vi "User_Info.vi"() -> ()   [LabVIEW 2020]
panel:
  in  "Change User":bool caption="切换用户"
  in  "User Manage":bool
  in  "Change Password":bool
  in  "User_Right":u16(ring) caption="权    限" items=["原厂管理员", "超级管理员", "操作者"]
  in  "User_Name":string caption="用户名"
  # "用户信息"
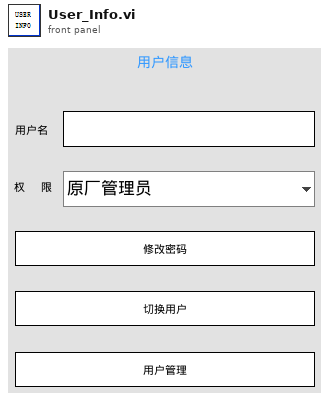
[diagram p1: front panel]
types:
  T1 = typedef "User_Info.ctl" = cluster{"Name":string, "Password":string, "User_Right":u16, "Debuger?":bool, "Manager?":bool, "User_Remember_Name":bool, "User_Remember_PW":bool, "User_Right_String":string, "Null?":bool, "Language":string}
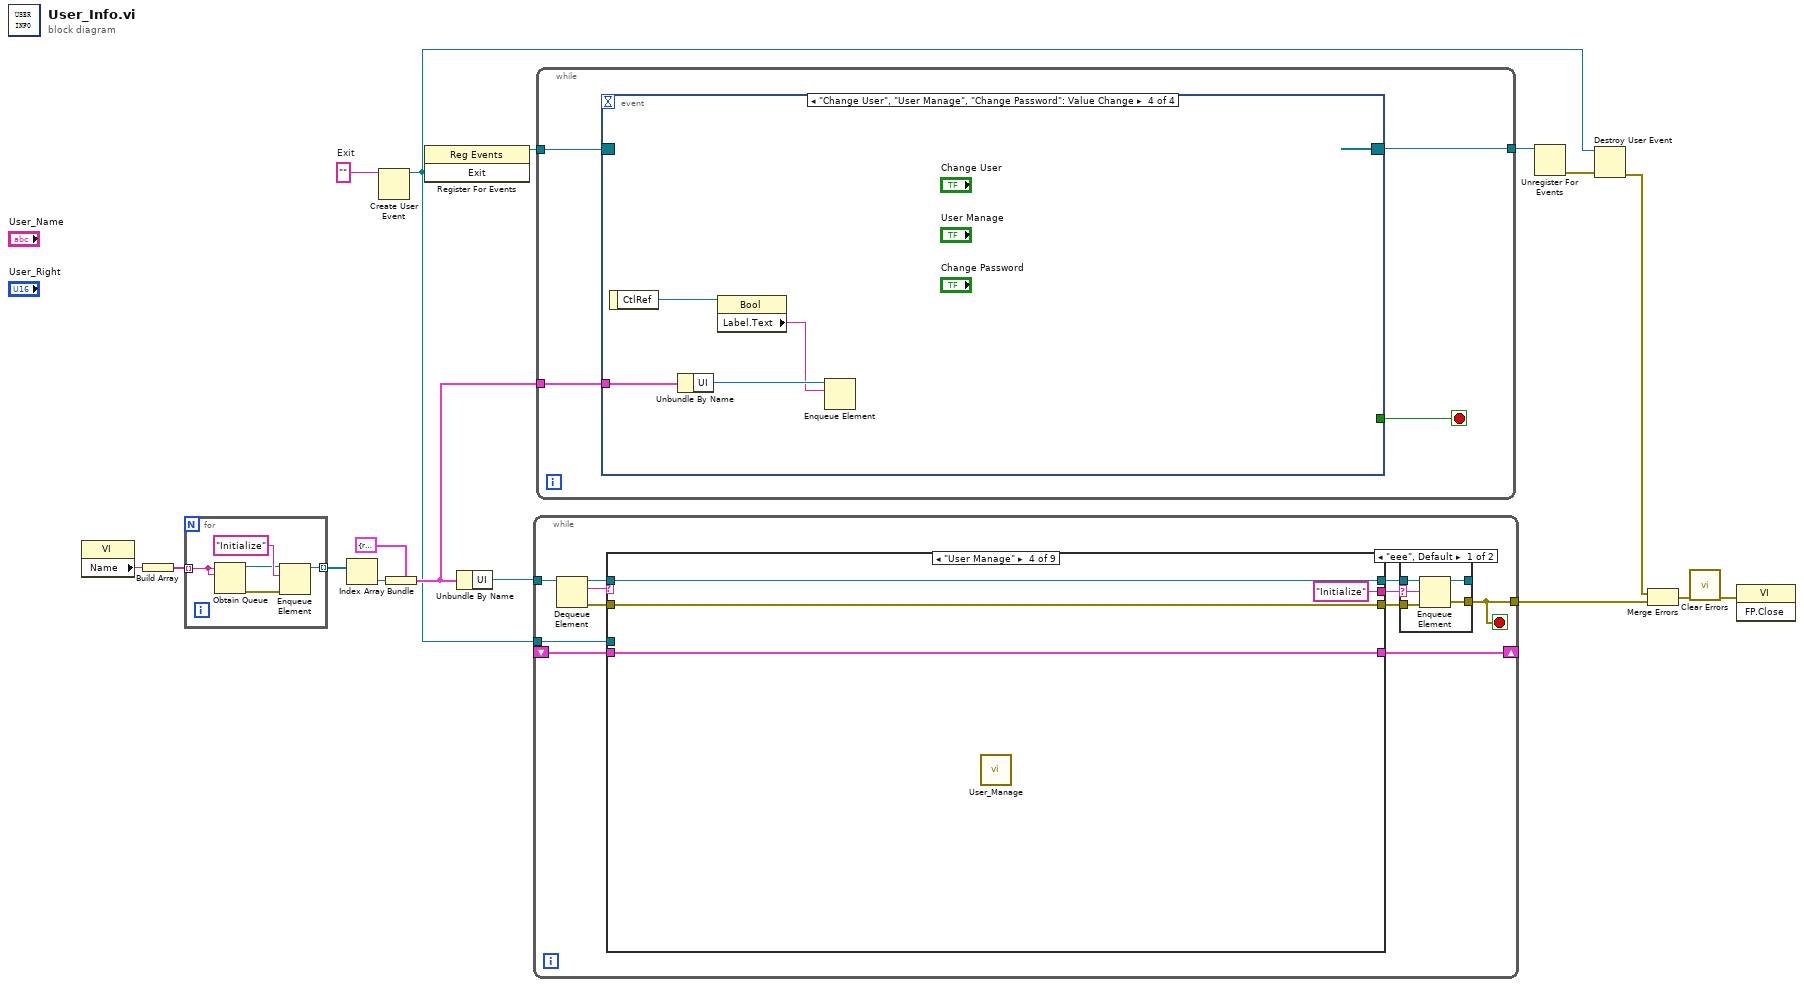
[diagram p0: block diagram]
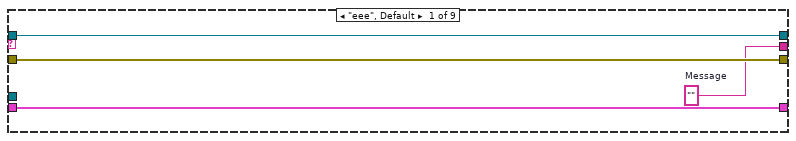
[diagram p3: hidden frame]
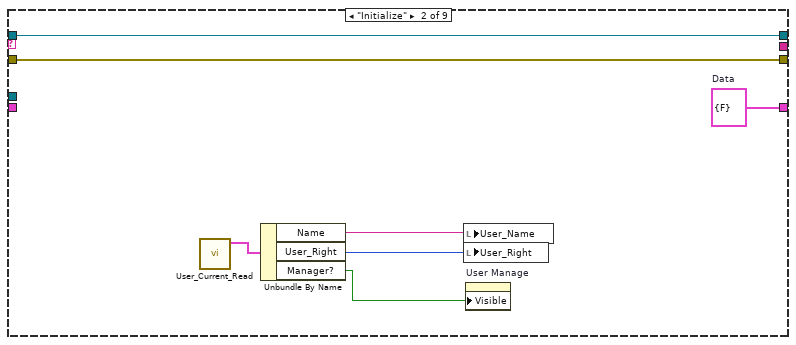
[diagram p4: hidden frame]
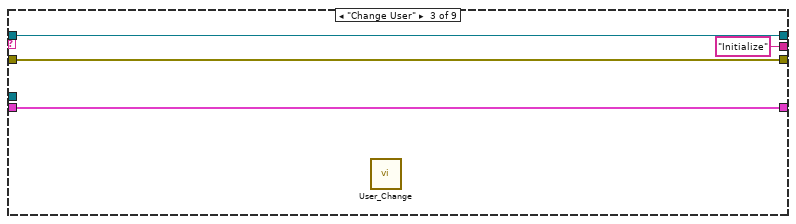
[diagram p5: hidden frame]
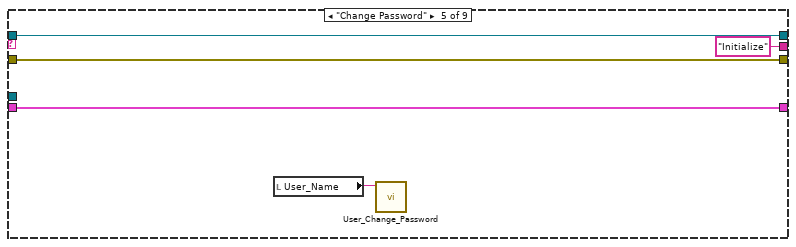
[diagram p6: hidden frame]
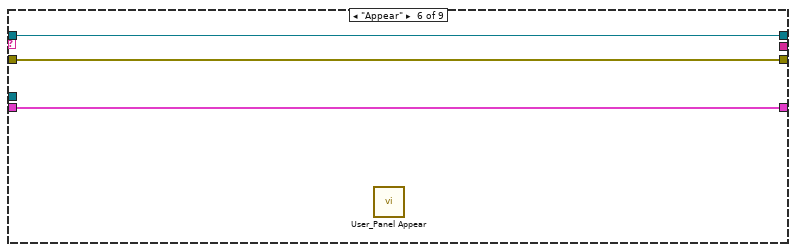
[diagram p7: hidden frame]
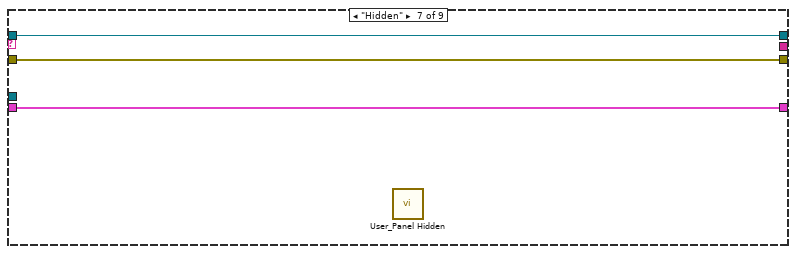
[diagram p8: hidden frame]
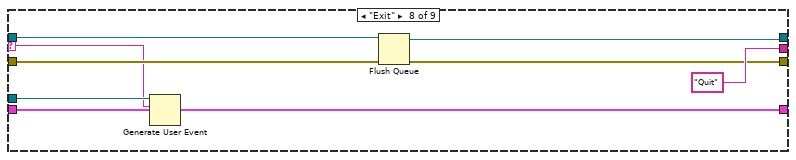
[diagram p9: hidden frame]
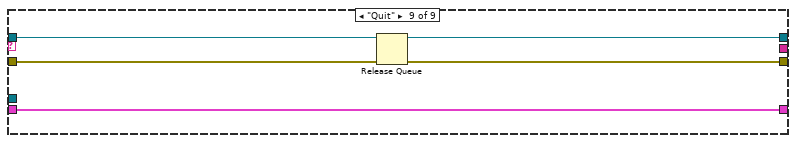
[diagram p10: hidden frame]
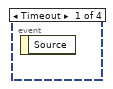
[diagram p11: hidden frame]
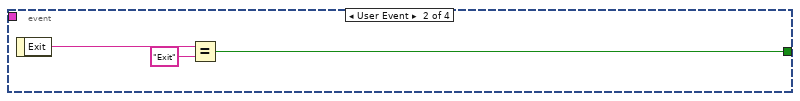
[diagram p12: hidden frame]
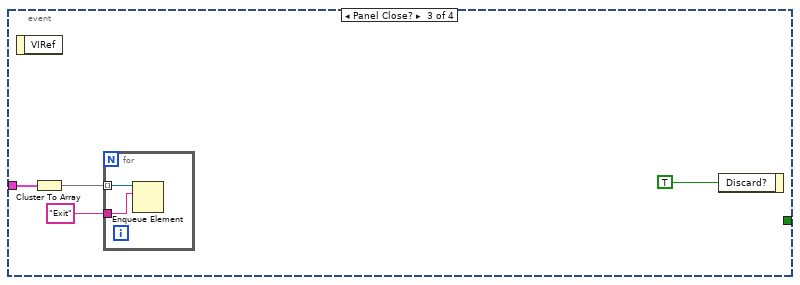
[diagram p13: hidden frame]
diagram:
  w2 = ""  # Exit
  n1 = property class="VI"() -> ("Name"=w12:string)  [unwired: 2 in, 2 out]
  n2 = Build Array(w12) -> (w13:string[])
  n3 = for {
    tunnel: w13 -> [w17] mode=indexing
    tunnel: [w18] -> w7 mode=indexing
    n4 = Obtain Queue(name (unnamed)=w17, element data type=w17) -> (queue out=w20:refnum<queue>, error out=w19:errorcluster)  [unwired: 3 in, 1 out]
    n5 = Enqueue Element(queue=w20, element="Initialize" ("元素"), error in (no error)=w19) -> (queue out=w18:refnum<queue>)  [unwired: 1 in, 2 out]
  }
  n6 = Index Array(array=w7) -> (element=w10:refnum<queue>)  [unwired: 1 in]
  n7 = Create User Event(user event datatype=w2) -> (user event=w6:refnum<user-event>)  [unwired: 1 in, 1 out]
  n8 = Bundle(cluster=cluster{"UI":refnum<queue>} {"UI"=refnum}, "UI"=w10) -> (w11:cluster{"UI":refnum<queue>})
  n9 = register-events(w6) -> (reference out=w3:refnum<event-registration>)  [unwired: 2 in, 1 out]
  n10 = Unbundle By Name(w11) -> ("UI"=w8:refnum<queue>)
  n11 = while {
    tunnel: w8 -> [w32]
    tunnel: [w22] -> w15
    shift-right: [w26] -> _
    shift-left: _ -> [w25]
    tunnel: w6 -> [w24]
    stop <- w22 stop-if-true
    n12 = Dequeue Element(queue=w32) -> (queue out=w31:refnum<queue>, element=w23:string, error out=w28:errorcluster)  [unwired: 2 in, 1 out]
    n13 = case shown="\"User Manage\"" w23 {
      selector: w23 -> [_ _ _ _ _ _ _ w70 _]
      tunnel: w31 -> [w43 w50 w54 w58 w63 w66 w69 w75 w81]
      tunnel: [w43 w50 w54 w58 w63 w66 w69 w74 w81] -> w30
      tunnel: [w42 w49 w53 w57 w62 w65 w68 w73 w78] -> w29
      tunnel: w28 -> [w42 w49 w53 w57 w62 w65 w68 w72 w80]
      tunnel: [w41 _ "Initialize" ("Message") "Initialize" ("Message") "Initialize" ("Message") _ _ "Quit" ("Message") _] -> w27
      tunnel: [w40 w48 w52 w56 w61 w64 w67 w77 w79] -> w26
      tunnel: w25 -> [w40 _ w52 w56 w61 w64 w67 w77 w79]
      tunnel: w24 -> [_ _ _ _ _ _ _ w71 _]
      frame "eee", Default {
        w41 = ""  # Message
      }
      frame "Initialize" {
        w48 = cluster{"Data":bool} {"Data"=FALSE}  # Data
        n14 = call "User_Current_Read.vi"() -> ("User_Info"=w47:T1)  [unwired: 10 in, 1 out]
        n15 = Unbundle By Name(w47) -> ("Name"=w46:string, "User_Right"=w45:u16, "Manager?"=w44:bool)
        n16 = local write "User_Name"(w46) -> ()
        n17 = local write "User_Right"(w45) -> ()
        n18 = property on="User Manage" class="Bool"("Visible"=w44) -> ()  [unwired: 2 in, 2 out]
      }
      frame "Change User" {
        n19 = call "User_Change.vi"() -> ()  [unwired: 12 in]
      }
      frame "User Manage" {
        n20 = call "User_Manage.vi"() -> ()  [unwired: 12 in]
      }
      frame "Change Password" {
        n21 = local read "User_Name"() -> (w59:string)
        n22 = call "User_Change_Password.vi"("User_Name"=w59) -> ()  [unwired: 11 in]
      }
      frame "Appear" {
        n23 = call "User_Panel Appear.vi"() -> ()  [unwired: 11 in, 1 out]
      }
      frame "Hidden" {
        n24 = call "User_Panel Hidden.vi"() -> ()  [unwired: 11 in, 1 out]
      }
      frame "Exit" {
        n25 = Generate User Event(user event=w71, event data cluster=w70) -> ()  [unwired: 2 in, 2 out]
        n26 = Flush Queue(queue=w75, error in (no error)=w72) -> (queue out=w74:refnum<queue>, error out=w73:errorcluster)  [unwired: 1 out]
      }
      frame "Quit" {
        n27 = Release Queue(queue=w81, error in (no error)=w80) -> (error out=w78:errorcluster)  [unwired: 1 in, 2 out]
      }
    }
    n28 = case shown="\"eee\", Default" w27 {
      selector: w27 -> [w33 _]
      tunnel: w30 -> [w37 w39]
      tunnel: w29 -> [w36 w38]
      tunnel: [w35 w38] -> w22
      tunnel: [w34 w39] -> _
      frame "eee", Default {
        n29 = Enqueue Element(queue=w37, element=w33, error in (no error)=w36) -> (queue out=w34:refnum<queue>, error out=w35:errorcluster)  [unwired: 1 in, 1 out]
      }
      frame "" {
      }
    }
  }
  n30 = while {
    tunnel: w3 -> [w84]
    tunnel: [w83] -> w5
    tunnel: w11 -> [w82]
    stop <- w85 stop-if-true
    n31 = event shown="[3] \"Change User\", \"User Manage\", \"Change Password\": Value Change" {
      selector: w84 -> [_ _ _ _]
      dyn-events: [_ _ _ _] -> w83
      timeout: _ -> [_ _ _ _]
      tunnel: [_ w87 _ _] -> w85
      tunnel: w82 -> [_ _ w91 w98]
      event Timeout {
        n32 = event-data() -> ()  [unwired: 1 in, 1 out]
      }
      event User Event {
        n33 = event-data() -> ("Exit"=w88:string)  [unwired: 1 in]
        n34 = Equal?(x=w88, y="Exit") -> (x = y?=w87:bool)
      }
      event Panel Close? {
        n35 = event-data() -> ()  [unwired: 1 in, 1 out]
        n36 = Cluster To Array(cluster=w91) -> (array=w90:refnum<queue>[])
        n37 = for {
          tunnel: w90 -> [w94] mode=indexing
          tunnel: "Exit" ("元素") -> [w93]
          n38 = Enqueue Element(queue=w94, element=w93) -> ()  [unwired: 2 in, 3 out]
        }
        n39 = event-data("Discard?"=TRUE ("放弃？")) -> ()  [unwired: 1 in, 1 out]
      }
      event "Change User", "User Manage", "Change Password": Value Change {
        n40 = event-data() -> ("CtlRef"=w96:refnum<vi>)  [unwired: 1 in]
        n41 = Unbundle By Name(w98) -> ("UI"=w97:refnum<queue>)
        n42 = property class="Bool"(reference=w96) -> ("Label.Text"=w95:string)  [unwired: 1 in, 2 out]
        n43 = Enqueue Element(queue=w97, element=w95) -> ()  [unwired: 2 in, 3 out]
      }
    }
  }
  n44 = Unregister For Events(event registration refnum=w5) -> (error out=w4:errorcluster)  [unwired: 1 in]
  n45 = Destroy User Event(user event=w6, error in=w4) -> (error out=w14:errorcluster)
  n46 = Merge Errors(w14, w15) -> (w16:errorcluster)
  n47 = call <vilib>:"Clear Errors.vi"("error in (no error)"=w16) -> ("error out"=w1:errorcluster)  [unwired: 5 in, 1 out]
  n48 = invoke class="VI" method="FP.Close"(error in=w1) -> ()  [unwired: 2 in, 3 out]
